vi "Undo.vi"(0 "reference in":refnum<class "PlayMusicCommand.lvclass">, 11 "Error In":errorcluster) -> (4 "reference out":refnum<class "PlayMusicCommand.lvclass">, 15 "Error Out":errorcluster)   [LabVIEW 2024, in "PlayMusicCommand.lvclass"]
doc: "Calls MediaPlayer and pauses music (opposite of play)."
uses:
  PlayMusicCommand.lvclass
  PlayMusicCommand.lvclass/PlayMusicCommand.ctl
  Receiver/MediaPlayer_class/MediaPlayer.lvclass
panel:
  # "Connector Pane"
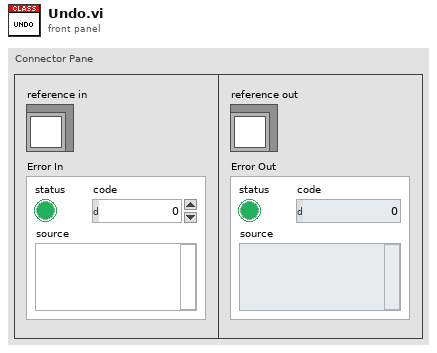
[diagram p1: front panel]
types:
  T1 = typedef "PlayMusicCommand.lvclass/ObjectAttributes.ctl" = cluster{"MediaPlayerRef":refnum<class "MediaPlayer.lvclass">}
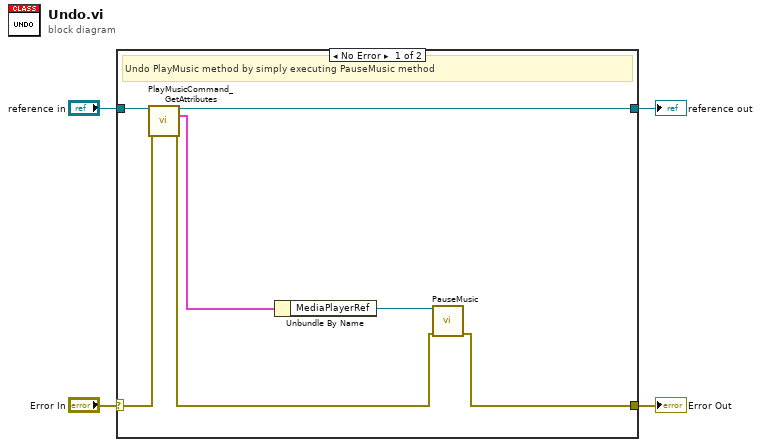
[diagram p0: block diagram]
diagram:
  n1 = case shown="No Error" "Error In" {
    selector: "Error In" -> [w11 w13]
    tunnel: [w5 w13] -> w3
    tunnel: [w8 w12] -> w1
    tunnel: "reference in" -> [w9 w12]
    frame No Error {
      # "Undo PlayMusic method by simply executing PauseMusic method"
      n2 = call "PlayMusicCommand_GetAttributes.vi"("reference in"=w9, "Error In"=w11) -> ("reference out"=w8:refnum<class "PlayMusicCommand.lvclass">, "Data"=w10:T1, "Error Out"=w6:errorcluster)  [unwired: 10 in, 1 out]
      n3 = Unbundle By Name(w10) -> ("MediaPlayerRef"=w7:refnum<class "MediaPlayer.lvclass">)
      n4 = call-dynamic "PauseMusic.vi"("reference in"=w7, "Error In"=w6) -> ("Error Out"=w5:errorcluster)  [unwired: 12 in, 1 out]
    }
    frame Error {
    }
  }
  "Error Out" <- w3
  "reference out" <- w1
